vi "Configure Control Mode.vi"(0 "VISA resource name":refnum<visa-resource-name>, 1 "Control Mode (0: Manual PID)":u16(ring) items=["Manual PID", "Zone", "Open Loop", "AutoTune PID", "AutoTune PI", "AutoTune P"], 2 "Setpoint Units (0: Kelvin)":u16(ring) items=["Kelvin", "Celsius", "Sensor Units"], 5 "Loop (0: 1)":u16(ring) items=["1", "2"], 7 "Input to \nControl From (0: A)":u16(ring) items=["A", "B"], 9 "Enable Powerup (F: OFF)":bool, 11 "error in (no error)":errorcluster, 12 "Heater Output Display (0: Current)":u16(ring) items=["Current", "Power"]) -> (4 "VISA resource name out":refnum<visa-resource-name>, 15 "error out":errorcluster)   [LabVIEW 2013, in "Lake Shore Cryotronics 331.lvlib"]
doc: "This VI selects a control loop's mode and configures the parameters of a control loop."
uses:
  Lake Shore Cryotronics 331.lvlib
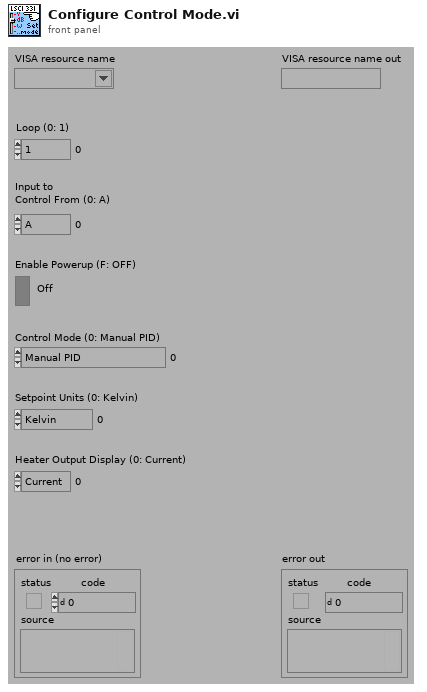
[diagram p1: front panel]
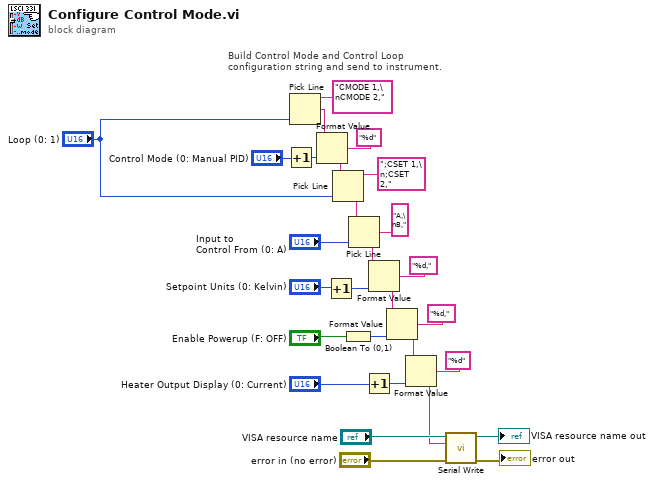
[diagram p0: block diagram]
diagram:
  # "Build Control Mode and Control Loop\nconfiguration string and send to instrument."
  n1 = Increment(x="Control Mode (0: Manual PID)") -> (x+1=w11:u16)
  n2 = Pick Line(multi-line string="CMODE 1,\nCMODE 2,", line index="Loop (0: 1)") -> (output string=w20:string)  [unwired: 1 in]
  n3 = Format Value(string ("")=w20, format string="%d", value (0)=w11) -> (output string=w19:string)
  n4 = Increment(x="Setpoint Units (0: Kelvin)") -> (x+1=w24:u16)
  n5 = Pick Line(string ("")=w19, multi-line string=";CSET 1,\n;CSET 2,", line index="Loop (0: 1)") -> (output string=w16:string)
  n6 = Boolean To (0,1)(Boolean="Enable Powerup (F: OFF)") -> (0, 1=w26:i16)
  n7 = Pick Line(string ("")=w16, multi-line string="A,\nB,", line index="Input to \nControl From (0: A)") -> (output string=w15:string)
  n8 = Increment(x="Heater Output Display (0: Current)") -> (x+1=w2:u16)
  n9 = Format Value(string ("")=w15, format string="%d,", value (0)=w24) -> (output string=w13:string)
  n10 = Format Value(string ("")=w13, format string="%d,", value (0)=w26) -> (output string=w12:string)
  n11 = Format Value(string ("")=w12, format string="%d", value (0)=w2) -> (output string=w4:string)
  n12 = call "Serial Write.vi"("error in (no error)"="error in (no error)", "Write Buffer (\"\")"=w4, "VISA resource name"="VISA resource name") -> ("error out"=→"error out":errorcluster, "VISA resource name out"=→"VISA resource name out":refnum<visa-resource-name>)  [unwired: 6 in, 1 out]
